vi "Read 1Chan NSamp 1D SGL.vi"(8 "error in (no error)":errorcluster, 9 "timeout [s]":dbl=-1.0, 10 "number of samples per channel":i32=1000, 11 "MicroDAQ.lvlib:Analog Input.lvclass":refnum<class "Analog Input.lvclass">) -> (0 "error out":errorcluster, 1 "read samples":i32, 2 "Values":dbl[](array[numeric]), 3 "MicroDAQ.lvlib:Analog Input.lvclass out":refnum<class "Analog Input.lvclass">)   [LabVIEW 2009, in "MicroDAQ.lvlib" / "Analog Input.lvclass"]
doc: "Reads a buffor of floating-point samples from a channel."
uses:
  <instrlib>/MicroDAQ/Channel/Analog Input/Analog Input.lvclass
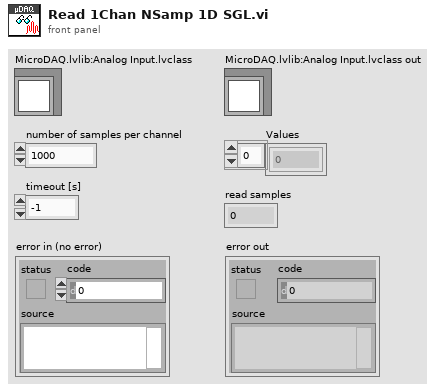
[diagram p1: front panel]
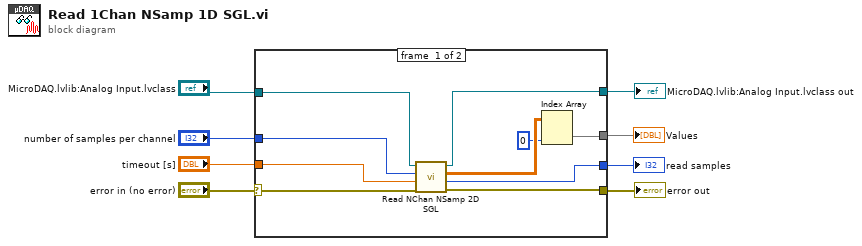
[diagram p0: block diagram]
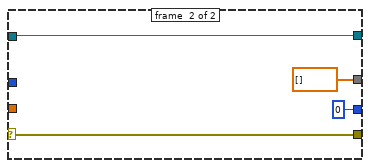
[diagram p2: hidden frame]
diagram:
  n1 = case shown="No Error" "error in (no error)" {
    selector: "error in (no error)" -> [w18 w21]
    tunnel: [w15 w21] -> w7
    tunnel: [w12 w22] -> w6
    tunnel: "MicroDAQ.lvlib:Analog Input.lvclass" -> [w17 w22]
    tunnel: [w14 dbl[] [] ("Values")] -> w4
    tunnel: "number of samples per channel" -> [w16 _]
    tunnel: [w11 0 ("read samples")] -> w2
    tunnel: "timeout [s]" -> [w9 _]
    frame #0 {
      n2 = call <instrlib>:"Read NChan NSamp 2D SGL.vi"("error in (no error)"=w18, "timeout [s]"=w9, "number of samples per channel"=w16, "MicroDAQ.lvlib:Analog Input.lvclass"=w17) -> ("error out"=w15:errorcluster, "read samples"=w11:i32, "Values"=w13:dbl[][], "MicroDAQ.lvlib:Analog Input.lvclass out"=w12:refnum<class "Analog Input.lvclass">)  [unwired: 4 in]
      n3 = Index Array(array=w13, index (col)=0 ("disabled index (col)")) -> (element=w14:dbl[])  [unwired: 1 in]
    }
    frame #1 {
    }
  }
  "error out" <- w7
  "MicroDAQ.lvlib:Analog Input.lvclass out" <- w6
  "Values" <- w4
  "read samples" <- w2
